vi "Update.vi"(8 "error in (no error)":errorcluster, 11 "Test Tree In":refnum<class "Test Tree.lvclass">) -> (0 "error out":errorcluster, 3 "Test Tree Out":refnum<class "Test Tree.lvclass">)   [LabVIEW 2020, in "Test Tree.lvclass"]
uses:
  Test Tree.lvclass
  Test Tree.lvclass/Test Tree.ctl
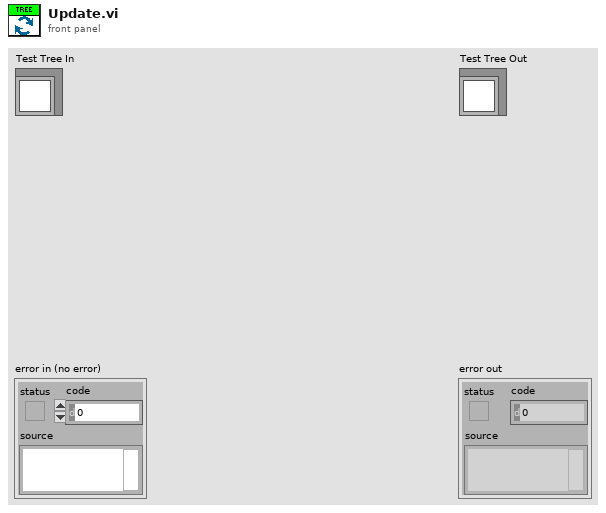
[diagram p1: front panel]
types:
  T1 = map{string, cluster{"Left Cell String":string, "Child Text":string[], "Item Indent":i32, "Child Only?":bool, "Glyph Index":i32}}
  T2 = cluster{"Left Cell String":string, "Child Text":string[], "Child Tag":string, "Item Indent":i32, "Child Only?":bool, "Glyph Index":i32}
  T3 = typedef "LVNodeAndColumnTypeDef.ctl" = cluster{"Node":string, "Column":i32}
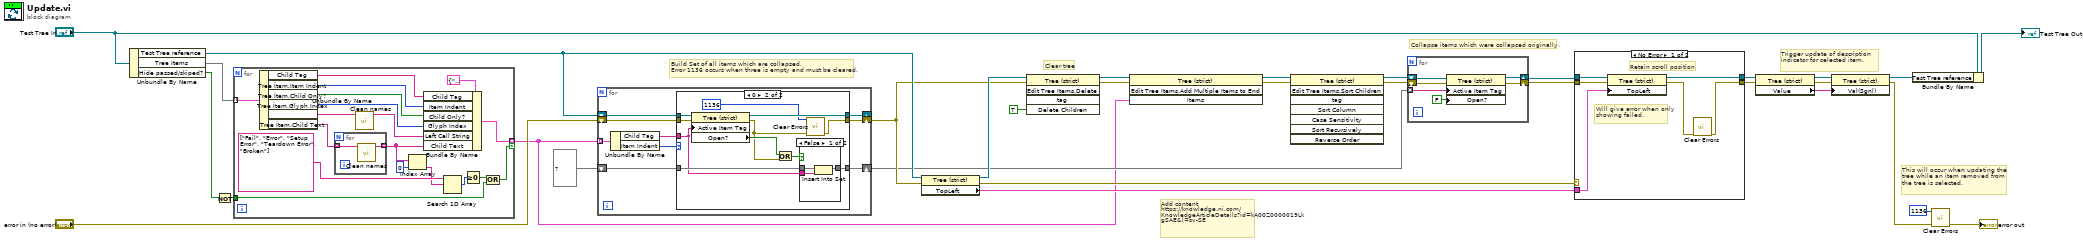
[diagram p0: block diagram]
diagram:
  # "Collapse items which were collapsed originally."
  # "Build Set of all items which are collapsed.\nError 1136 occurs when three is empty and must be cleared."
  # "This will occur when updating the tree while an item removed from the tree is selected."
  # "Trigger update of description indicator for selected item."
  # "Add content\nhttps://knowledge.ni.com/KnowledgeArticleDetails?id=kA00Z0000019LkgSAE&l=sv-SE"
  # "Clear tree"
  n1 = Unbundle By Name("Test Tree In") -> ("Test Tree reference"=w15:refnum<vi>, "Tree Items"=w26:T1, "Hide passed/skiped?"=w1:bool)
  n2 = Not(x=w1) -> (.not. x?=w27:bool)
  n3 = for {
    tunnel: w26 -> [w50] mode=indexing
    tunnel: [w49] -> w2 mode=indexing if=w42
    tunnel: w27 -> [w43]
    n4 = Unbundle By Name(w50) -> ("Child Tag"=w33:string, "Tree Ítem.Item Indent"=w34:i32, "Tree Ítem.Child Only?"=w35:bool, "Tree Ítem.Glyph Index"=w36:i32, "Tree Ítem.Left Cell String"=w48:string, "Tree Ítem.Child Text"=w47:string[])
    n5 = for {
      tunnel: [w52] -> w45 mode=indexing
      tunnel: w47 -> [w51] mode=indexing
      n6 = call "Clean names.vi"("Name with extension"=w51) -> ("Name without extension"=w52:string)  [unwired: 10 in]
    }
    n7 = call "Clean names.vi"("Name with extension"=w48) -> ("Name without extension"=w46:string)  [unwired: 10 in]
    n8 = Index Array(array=w45, index=0) -> (element=w40:string)
    n9 = Bundle By Name(cluster=T2 {"Left Cell String"="", "Child Text"=[], "Child Tag"="", "Item Indent"=0, "Child Only?"=FALSE, "Glyph Index"=0} ("Item"), "Child Tag"=w33, "Item Indent"=w34, "Child Only?"=w35, "Glyph Index"=w36, "Left Cell String"=w46, "Child Text"=w45) -> (w49:T2)
    n10 = Search 1D Array(1D array=string[] ["Fail", "Error", "Setup Error", "Teardown Error", "Broken"] ("y"), element=w40) -> (index of element=w39:i32)  [unwired: 1 in]
    n11 = Greater Or Equal To 0?(x=w39) -> (x >= 0?=w38:bool)
    n12 = Compound Arithmetic op=OR(w38, w43) -> (w42:bool)
  }
  n13 = for {
    tunnel: w2 -> [w61] mode=indexing
    shift-right: [w59] -> _
    shift-left: w15 -> [w60]
    shift-right: [w54] -> w13
    shift-left: "error in (no error)" -> [w55]
    shift-right: [w57] -> w11
    shift-left: set{string} {} ("set") -> [w58]
    n14 = Unbundle By Name(w61) -> ("Child Tag"=w56:string, "Item Indent"=w53:i32)
    n15 = case shown="0" w53 {
      tunnel: w60 -> [w63 w75]
      tunnel: [w63 w74] -> w59
      tunnel: w58 -> [w64 w73]
      tunnel: [w64 w72] -> w57
      tunnel: w56 -> [_ w71]
      tunnel: w55 -> [w62 w69]
      tunnel: [w62 w68] -> w54
      frame Default {
      }
      frame 0 {
        n16 = property class="Tree (strict)"(reference=w75, error in=w69, "Active Item Tag"=w71) -> (reference out=w74:refnum<vi>, error out=w65:errorcluster, "Open?"=w70:bool)
        n17 = Or(x=w70, y=w65) -> (x .or. y?=w66:bool)
        n18 = case shown="False" w66 {
          tunnel: w73 -> [w78 w79]
          tunnel: [w77 w79] -> w72
          tunnel: w71 -> [w76 _]
          frame False {
            n19 = Insert Into Set(10:w76, 11:w78) -> (3:w77:set{string})  [unwired: 1 out]
          }
          frame True {
          }
        }
        n20 = call <vilib>:"Clear Errors.vi"("error in (no error)"=w65, "specific error code to clear (0: all)"=1136) -> ("error out"=w68:errorcluster)  [unwired: 4 in, 1 out]
      }
    }
  }
  n21 = property on="Property Node" class="Tree (strict)"(reference=w15, error in=w13) -> (reference out=w25:refnum<vi>, error out=w24:errorcluster, "TopLeft"=w23:T3)
  n22 = invoke on="Invoke Node" class="Tree (strict)" method="Edit Tree Items.Delete"(reference=w25, error in=w13, "Delete Children"=TRUE ("Delete Children?")) -> (reference out=w29:refnum<vi>, error out=w28:errorcluster)  [unwired: 2 in, 3 out]
  n23 = invoke class="Tree (strict)" method="Edit Tree Items.Add Multiple Items to End"(reference=w29, error in=w28, "Items"=w2) -> (reference out=w8:refnum<vi>, error out=w4:errorcluster)  [unwired: 1 in, 2 out]
  n24 = invoke class="Tree (strict)" method="Edit Tree Items.Sort Children"(reference=w8, error in=w4) -> (reference out=w5:refnum<vi>, error out=w3:errorcluster)  [unwired: 6 in, 6 out]
  n25 = for {
    shift-right: [w84] -> w7
    shift-left: w5 -> [w85]
    shift-right: [w83] -> w6
    shift-left: w3 -> [w82]
    tunnel: w11 -> [w81] mode=indexing
    n26 = property class="Tree (strict)"(reference=w85, error in=w82, "Active Item Tag"=w81, "Open?"=FALSE ("Active Item:Open?")) -> (reference out=w84:refnum<vi>, error out=w83:errorcluster)
  }
  n27 = case shown="No Error" w24 {
    tunnel: w7 -> [w91 w93]
    tunnel: [w90 w93] -> w10
    tunnel: w6 -> [w89 w92]
    tunnel: [w86 w92] -> w9
    tunnel: w23 -> [w87 _]
    frame No Error {
      # "Will give error when only showing failed."
      # "Retain scroll position"
      n28 = property on="Property Node" class="Tree (strict)"(reference=w91, error in=w89, "TopLeft"=w87) -> (reference out=w90:refnum<vi>, error out=w88:errorcluster)
      n29 = call <vilib>:"Clear Errors.vi"("error in (no error)"=w88) -> ("error out"=w86:errorcluster)  [unwired: 5 in, 1 out]
    }
    frame Error {
      # "There is nothing in the tree, so the top left will return error."
    }
  }
  n30 = property on="Property Node" class="Tree (strict)"(reference=w10, error in=w9) -> (reference out=w22:refnum<vi>, error out=w21:errorcluster, "Value"=w18:string[])
  n31 = property on="Property Node" class="Tree (strict)"(reference=w22, error in=w21, "Val(Sgnl)"=w18) -> (reference out=w20:refnum<vi>, error out=w19:errorcluster)
  n32 = Bundle By Name(cluster="Test Tree In", "Test Tree reference"=w20) -> (→"Test Tree Out":refnum<class "Test Tree.lvclass">)
  n33 = call <vilib>:"Clear Errors.vi"("error in (no error)"=w19, "specific error code to clear (0: all)"=1136) -> ("error out"=→"error out":errorcluster)  [unwired: 4 in, 1 out]
